vi "Get Document With Where.vi"(8 "error in (no error)":errorcluster caption="entrée d'erreur (pas d'erreur)", 11 "Firebase (Default) en entrée":refnum<class "Firebase Driver.lvclass">) -> (0 "error out":errorcluster caption="sortie d'erreur", 3 "Firebase (Default) en sortie":refnum<class "Firebase Driver.lvclass">)   [LabVIEW 2020, in "Library Instrument & Equipement.lvlib" / "Library FireBase.lvlib" / "Firebase Driver.lvclass"]
uses:
  Firebase Driver.lvclass
  Commun VI/TypeDef/Liste Error.ctl
  Firebase Driver.lvclass/Firebase Driver.ctl
  <vilib>/httpClient/POSTBuffer.vi
  <vilib>/httpClient/LabVIEWHTTPClient.lvlib
  Commun VI/Library Commun.lvlib
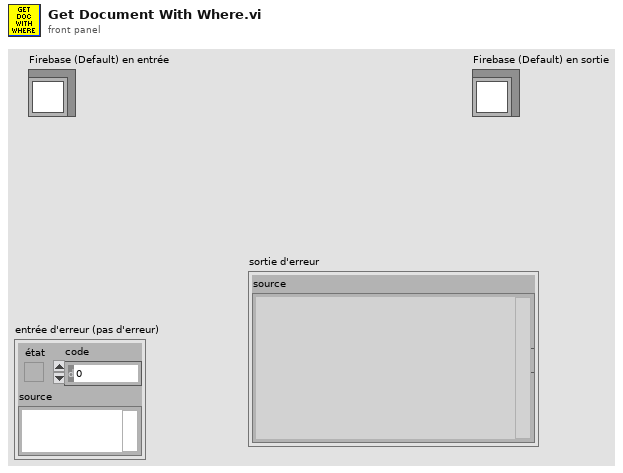
[diagram p1: front panel]
types:
  T1 = typedef "Library Commun.lvlib/Liste Error.ctl" = enum16{"Firebase Driver - Get Document", "Firebase Driver - Get Document With Where", "Firebase Driver - Delete Document", "Firebase Driver - Set Document", "Firebase Driver - Update Document", "Firebase Altyor - Search Document Bench", "Firebase Altyor - Class Not in Firebase", "Spectrum_Analyser - Timeout", "Relay Board - Qty Relay", "DIO - Pb Funtion", "Power_Supply - Peripherical not find", "Mutimeter - Peripherical not find", "Instrument - Function Not Used", "Instrument - Instrument name not specified", "Instrument - Allready Initialised", "Instrument - TimeOut", "Instrument - the instrument must be Initialise before", "Instrument - Frame Not received", "Instrument - Frame Nok", "Test - Initialise the File_for_Save", "Test - Timeout", "Test - Cmd Error", "FGV - Variable ", "BDD FireBase - Define Class", "SN - Class Not Define"}
  T2 = typedef "LabVIEWHTTPClient.lvlib/ClientHandle.ctl" = refnum<k1>
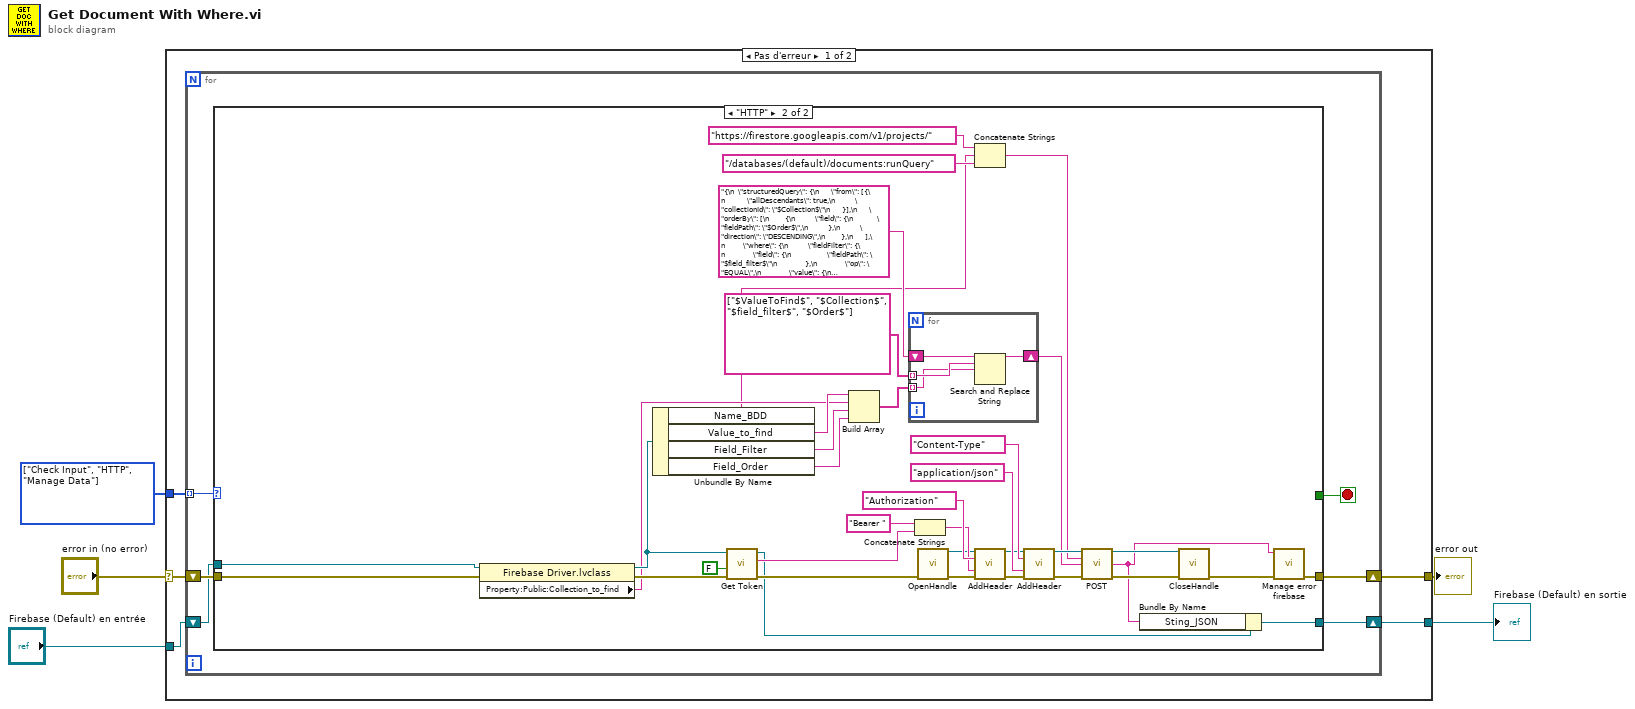
[diagram p0: block diagram]
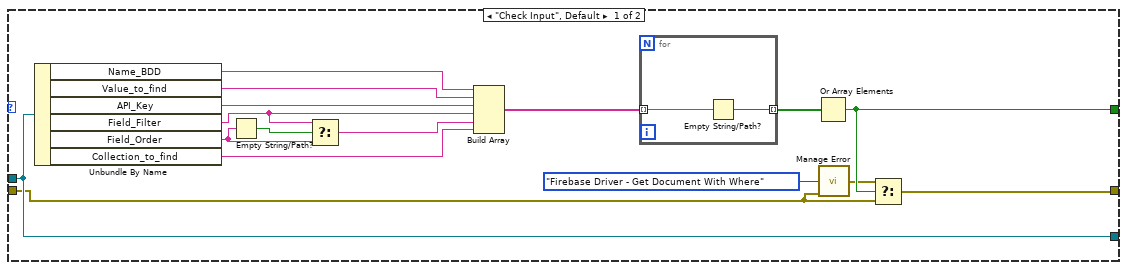
[diagram p2: hidden frame]
diagram:
  w1 = enum16{"Check Input", "HTTP", "Manage Data"}[] [enum."Check Input", enum."HTTP", enum."Manage Data"] items=["Check Input", "HTTP", "Manage Data"]
  n1 = case shown="Pas d'erreur" "error in (no error)" {
    selector: "error in (no error)" -> [w10 w77]
    tunnel: [w9 w77] -> w4
    tunnel: "Firebase (Default) en entrée" -> [w8 w76]
    tunnel: [w7 w76] -> w2
    tunnel: w1 -> [w6 _]
    frame No Error {
      n2 = for {
        shift-right: [w13] -> w9
        shift-left: w10 -> [w16]
        shift-right: [w14] -> w7
        shift-left: w8 -> [w15]
        tunnel: w6 -> [w12] mode=indexing
        stop <- w11 stop-if-true
        n3 = case shown="\"HTTP\"" w12 {
          tunnel: w16 -> [w17 w38]
          tunnel: w15 -> [w32 w41]
          tunnel: [w32 w47] -> w14
          tunnel: [w26 w48] -> w13
          tunnel: [w27 _] -> w11
          frame "Check Input", Default {
            n4 = Unbundle By Name(w32) -> ("Name_BDD"=w31:string, "Value_to_find"=w30:string, "API_Key"=w25:string, "Field_Filter"=w23:string, "Field_Order"=w21:string, "Collection_to_find"=w20:string)
            n5 = Empty String/Path?(string/path=w21) -> (empty?=w24:bool)
            n6 = Select(t=w23, s=w24, f=w21) -> (s? t:f=w22:string)
            n7 = Build Array(w31, w30, w25, w23, w22, w20) -> (w29:string[])
            n8 = for {
              tunnel: w29 -> [w34] mode=indexing
              tunnel: [w33] -> w28 mode=indexing
              n9 = Empty String/Path?(string/path=w34) -> (empty?=w33:bool)
            }
            n10 = Or Array Elements(Boolean array=w28) -> (logical OR=w27:bool)
            n11 = call "Manage Error.vi"("Code Erreur"=Liste_Error."Firebase Driver - Get Document With Where", "error in (no error)"=w17) -> ("error out"=w19:errorcluster)  [unwired: 13 in]
            n12 = Select(t=w19, s=w27, f=w17) -> (s? t:f=w26:errorcluster)
          }
          frame "HTTP" {
            n13 = property class="Firebase Driver.lvclass"(reference=w41, error in=w38) -> (reference out=w40:refnum<class "Firebase Driver.lvclass">, error out=w39:errorcluster, "Property:Public:Collection_to_find"=w37:string)
            n14 = Unbundle By Name(w40) -> ("Name_BDD"=w36:string, "Value_to_find"=w49:string, "Field_Filter"=w42:string, "Field_Order"=w43:string)
            n15 = call-dynamic "Get Token.vi"("error in (no error)"=w39, "Reset"=FALSE, "Build Library FireBase.lvlib:Firebase (Default) IN"=w40) -> ("error out"=w57:errorcluster, "idToken"=w45:string, "Build Library FireBase.lvlib:Firebase (Default) Out"=w44:refnum<class "Firebase Driver.lvclass">)  [unwired: 6 in]
            n16 = Build Array(w49, w37, w42, w43) -> (w50:string[])
            n17 = for {
              shift-right: [w74] -> w55
              shift-left: "{\n  \"structuredQuery\": {\n      \"from\": [{\n           \"allDescendants\": true,\n          \"collectionId\": \"$Collection$\"\n      }],\n      \"orderBy\": [\n        {\n          \"field\": {\n            \"fieldPath\": \"$Order$\",\n          },\n          \"direction\": \"DESCENDING\",\n        },\n      ],\n         \"where\": {\n          \"fieldFilter\": {\n              \"field\": {\n                  \"fieldPath\": \"$field_filter$\"\n              },\n              \"op\": \"EQUAL\",\n              \"value\": {\n                  stringValue: \"$ValueToFind$\"\n              }\n          }\n      }\n  }\n}" -> [w75]
              tunnel: string[] ["$ValueToFind$", "$Collection$", "$field_filter$", "$Order$"] -> [w73] mode=indexing
              tunnel: w50 -> [w72] mode=indexing
              n18 = Search and Replace String(input string=w75, search string=w73, replace string=w72) -> (result string=w74:string)  [unwired: 5 in, 3 out]
            }
            n19 = Concatenate Strings("Bearer " ("chaîne"), w45) -> (w63:string)
            n20 = call <vilib>:"OpenHandle.vi"("error in (no error)"=w57) -> ("client handle out"=w62:T2, "error out"=w60:errorcluster)  [unwired: 13 in]
            n21 = Concatenate Strings("https://firestore.googleapis.com/v1/projects/" ("string"), w36, "/databases/(default)/documents:runQuery" ("string")) -> (w52:string)
            n22 = call <vilib>:"AddHeader.vi"("client handle"=w62, "header"="Authorization", "value"=w63, "error in (no error)"=w60) -> ("client handle out"=w66:T2, "error out"=w67:errorcluster)  [unwired: 10 in]
            n23 = call <vilib>:"AddHeader.vi"("client handle"=w66, "header"="Content-Type", "value"="application/json", "error in (no error)"=w67) -> ("client handle out"=w61:T2, "error out"=w59:errorcluster)  [unwired: 10 in]
            n24 = call-poly <vilib>:"POST.vi"("client handle"=w61, "url"=w52, "buffer"=w55, "error in (no error)"=w59) -> ("client handle out"=w71:T2, "body"=w46:string, "error out"=w70:errorcluster)  [unwired: 8 in, 1 out]
            n25 = Bundle By Name(cluster=w44, "Sting_JSON"=w46) -> (w47:refnum<class "Firebase Driver.lvclass">)
            n26 = call <vilib>:"CloseHandle.vi"("client handle"=w71, "error in (no error)"=w70) -> ("error out"=w58:errorcluster)  [unwired: 13 in]
            n27 = call "Manage error firebase.vi"("error in (no error)"=w58, "Body"=w46) -> ("error out"=w48:errorcluster)  [unwired: 9 in]
          }
        }
      }
    }
    frame Error {
    }
  }
  "error out" <- w4
  "Firebase (Default) en sortie" <- w2
